vi "EnFlo_Hub.vi"() -> ()   [LabVIEW 2012]
uses:
  Anemometry Sub Vis/Controls/Launch_controls/Open_Calib.ctl
  Anemometry Sub Vis/Controls/Launch_controls/Open_Meas.ctl
  Anemometry Sub Vis/Controls/Launch_controls/Open_Enter_Temp.ctl
  Anemometry Sub Vis/Controls/Launch_controls/Multi_Run_Prog.ctl
  Anemometry Sub Vis/Controls/Launch_controls/EnFlo_arm.ctl
  Anemometry Sub Vis/Controls/Launch_controls/Fast_FID_Valve.ctl
  Anemometry Sub Vis/Controls/Launch_controls/Disp_Setup.ctl
  Anemometry Sub Vis/Controls/Launch_controls/EnFlo_Tun_Setup.ctl
  Anemometry Sub Vis/Controls/Launch_controls/User_Metadata.ctl
  Anemometry Sub Vis/Controls/Launch_controls/Trav_3D_move.ctl
  Anemometry Sub Vis/Controls/Launch_controls/Trav_Space.ctl
  Anemometry Sub Vis/Controls/Launch_controls/Tunnel_speed.ctl
  Anemometry Sub Vis/Controls/Launch_controls/Client_source_control.ctl
  Anemometry Sub Vis/Controls/Launch_controls/Hydrosonic_Manual.ctl
  Anemometry Sub Vis/Controls/Launch_controls/Preference_Panel.ctl
  Anemometry Sub Vis/Controls/Launch_controls/Hot_wire_Calculator.ctl
  Anemometry Sub Vis/Controls/Launch_controls/RW_X_Parker_Config.ctl
  Anemometry Sub Vis/Controls/Launch_controls/LDA_Alignment.ctl
  Anemometry Sub Vis/Controls/Launch_controls/Named_Serial_Comms.ctl
  Anemometry Sub Vis/Controls/Launch_controls/BSA_data_rates.ctl
  Anemometry Sub Vis/Controls/Launch_controls/Serial_Setup.ctl
  Anemometry Sub Vis/Controls/Launch_controls/Post_Process_icon.ctl
  Anemometry Sub Vis/Controls/Launch_controls/Edit_Ascii_file.ctl
  Anemometry Sub Vis/Controls/Launch_controls/Edit_Raw_DF.ctl
  Anemometry Sub Vis/Controls/Launch_controls/Results_file_plotter.ctl
  Anemometry Sub Vis/Controls/Launch_controls/Serial_Port_Names.ctl
  Anemometry Sub Vis/Controls/Launch_controls/Paul.ctl
  Anemometry Sub Vis/Controls/Launch_controls/Tom.ctl
  Anemometry Sub Vis/Controls/Launch_controls/Scani_Valve.ctl
  Anemometry Sub Vis/Controls/Launch_controls/Edit_sever_Channel.ctl
  Anemometry Sub Vis/Controls/Launch_controls/Day_file_plotter.ctl
  Anemometry Sub Vis/Controls/Launch_controls/Plot_Sever_Data.ctl
  Anemometry Sub Vis/Controls/Launch_controls/Adam_Table.ctl
  Anemometry Sub Vis/Controls/Launch_controls/Active_Channel_Control.ctl
  Anemometry Sub Vis/Controls/Setup.ctl
  Anemometry Sub Vis/Controls/Post_Process.ctl
  Anemometry Sub Vis/Controls/Preference_Mode.ctl
  Anemometry Sub Vis/Gen Trav/Trav_mode.ctl
  Anemometry Sub Vis/Controls/User_Specific_mode.ctl
  Anemometry Sub Vis/File/Setup_Filetype.ctl
  Anemometry Sub Vis/Calibration/Calib_mode.ctl
  Anemometry Sub Vis/Controls/Server_Comms.ctl
  Anemometry Sub Vis/Controls/App_Global.ctl
  Anemometry Sub Vis/Globals/Dynamic_call_global.ph.vi
  Anemometry Sub Vis/Globals/Constants_global.vi
  Anemometry Sub Vis/Globals/Preference_global.vi
  Anemometry Sub Vis/Globals/Meas_global.vi
  <vilib>/Platform/browser.llb/Open URL in Default Browser (string).vi
  Anemometry Sub Vis/Globals/Trav_pos_global.vi
  Anemometry Sub Vis/Acquisition/PWA/PWAtasksGLOBAL.vi
  Anemometry Sub Vis/Utilities/Email_transfer_global.vi
panel:
  out "List of ADAM channels to view":string[](array[string])
  out "List of ADAM control channels":string[](array[string])
  out "Analogue Dev Name":string="Dev2"
  out "Numeric":i32
  out "Rig Name":string="EnFlo Tunnel"
  out "All Users":path=path "/System Folder/Preferences/LabVIEW (EnFlo specific)/Meas Setups"
  out "Dummy Measurement":bool
  in  "stop":bool
  in  "Tab Control":T1(tab)
  in  "Tunnel Speed Control":T2
  in  "Traverse Space":T3
  in  "Trav 3D Move":T4 caption="3D Traverse Move"
  in  "User Metadata":T5
  in  "Multi Run Prog":T6
  in  "Enter Temp_Press":T7
  in  "Measurement Prog":T8 caption="Measurement"
  in  "Calibration Prog":T9 caption="Calibration"
  in  "Scani Valve":T10
  in  "LDA Alignment":T11
  in  "Hydrosonic Control":T12
  in  "Fast FID Valve":T13
  in  "Source Control":T14
  in  "Gas Release Setup":T15
  in  "EnFlo Tunnel Setup":T16
  in  "Heater Setup":bool caption="Inlet heater File"
  in  "EnFlo Arm":T17
  in  "EnFlo Tun Display":bool
  in  "Rig_Control":cluster{"Ch Name":string, "Boolean":bool}[](array[cluster])
  in  "ADAM Channels Control":T18 caption="Change Active Channels"
  in  "ADAM Scan Table":T19 caption="Run ADAM Scan Table"
  in  "Edit Server Channel":T20
  in  "Plot Server Channels":T21 caption="Plot Server Data"
  in  "Day Files Plotter":T22 caption="Plot Data From File"
  out "Current Values":cluster{"Ch Name":string, "Numeric":dbl}[](array[cluster])
  in  "Results File Plotter":T23
  in  "Edit Raw Data Files":T24
  in  "Edit ASCII File":T25
  in  "Post Process Raw Data":T26
  in  "Port Names":T27
  in  "Serial Setup":T28
  in  "LDA Data Rate":T29
  in  "Named Serial Comms":T30
  in  "RW Trav Setup":T31
  in  "Hot Wire Calc":T32
  in  "Preference Panel":T33
  in  "Tom Lawton t.lawton@surrey.ac.uk":T34 caption="For hardware support"
  in  "Paul Hayden p.hayden@surrey.ac.uk":T35 caption="For software support"
  in  "Online Manual":bool
  out "VI Name":string
  out "Iterations":i32
  # "Or give us a call on Tel: 01483 689545"
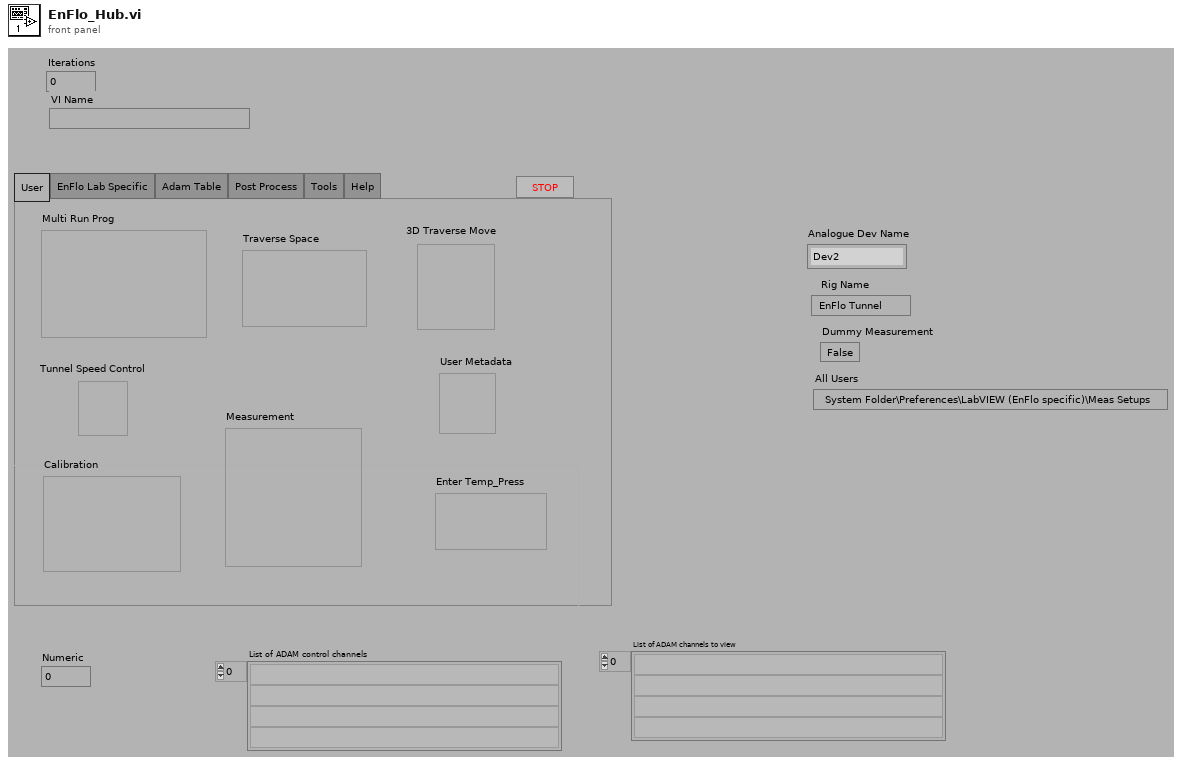
[diagram p1: front panel]
types:
  T1 = enum32{"User", "EnFlo Lab Specific", "Adam Table", "Post Process", "Tools", "Help"}
  T2 = typedef "Tunnel_speed.ctl" = bool
  T3 = typedef "Trav_Space.ctl" = bool
  T4 = typedef "Trav_3D_move.ctl" = bool
  T5 = typedef "User_Metadata.ctl" = bool
  T6 = typedef "Multi_Run_Prog.ctl" = bool
  T7 = typedef "Open_Enter_Temp.ctl" = bool
  T8 = typedef "Open_Meas.ctl" = bool
  T9 = typedef "Open_Calib.ctl" = bool
  T10 = typedef "Scani_Valve.ctl" = bool
  T11 = typedef "LDA_Alignment.ctl" = bool
  T12 = typedef "Hydrosonic_Manual.ctl" = bool
  T13 = typedef "Fast_FID_Valve.ctl" = bool
  T14 = typedef "Client_source_control.ctl" = bool
  T15 = typedef "Disp_Setup.ctl" = bool
  T16 = typedef "EnFlo_Tun_Setup.ctl" = bool
  T17 = typedef "EnFlo_arm.ctl" = bool
  T18 = typedef "Active_Channel_Control.ctl" = bool
  T19 = typedef "Adam_Table.ctl" = bool
  T20 = typedef "Edit_sever_Channel.ctl" = bool
  T21 = typedef "Plot_Sever_Data.ctl" = bool
  T22 = typedef "Day_file_plotter.ctl" = bool
  T23 = typedef "Results_file_plotter.ctl" = bool
  T24 = typedef "Edit_Raw_DF.ctl" = bool
  T25 = typedef "Edit_Ascii_file.ctl" = bool
  T26 = typedef "Post_Process_icon.ctl" = bool
  T27 = typedef "Serial_Port_Names.ctl" = bool
  T28 = typedef "Serial_Setup.ctl" = bool
  T29 = typedef "BSA_data_rates.ctl" = bool
  T30 = typedef "Named_Serial_Comms.ctl" = bool
  T31 = typedef "RW_X_Parker_Config.ctl" = bool
  T32 = typedef "Hot_wire_Calculator.ctl" = bool
  T33 = typedef "Preference_Panel.ctl" = bool
  T34 = typedef "Tom.ctl" = bool
  T35 = typedef "Paul.ctl" = bool
  T36 = typedef "Post_Process.ctl" = enum16{"Take New Data", "Post Process Raw Data File"}
  T37 = typedef "Setup.ctl" = enum16{"Run Program", "Show Setup", "Save Current Setup", "Setup Front Panel"}
  T38 = enum16{"Get Channel Names", "Get Current Value", "Update Channel Value", "Update Channel Description"}
  T39 = enum32{"Invalid", "Standard", "Closed", "Hidden", "Minimized", "Maximized"}
  T40 = typedef "Preference_Mode.ctl" = enum16{"Load Preferences from file", "Save Preferences to file", "Load, Edit then Save"}
  T41 = typedef "User_Specific_mode.ctl" = enum16{"Check VI only", "Run VI"}
  T42 = typedef "Trav_mode.ctl" = enum16{"Move traverse", "Read traverse position", "Teach Position"}
  T43 = typedef "Setup_Filetype.ctl" = enum16{"Measurement Setups", "Calibration Setups", "General", "Results File Plotter Setups", "Speed Calib Tweaks"}
  T44 = enum16{"Load Command File", "Save Command File", "Check Multi Run Prog", "Check Multi Run Prog With Live Moves", "Run Multi Run Prog"}
  T45 = typedef "Calib_mode.ctl" = enum16{"Show Setup", "Take a New Calibration Point", "Refit Curve", "Setup Front Panel"}
  T46 = typedef "Tunnel_Coordinates.ctl" = enum16{"Work in Tunnel Coordinates", "Work in Model Coordinates"}
  T47 = typedef "App_Global.ctl" = enum16{"Read Global", "Write to Global", "Initialise Array"}
  T48 = typedef "App_Ref_Cluster.ctl" = cluster{"Server IP & Port No":string, "Application reference":refnum<vi>}
  T49 = typedef "Server_Comms.ctl" = enum16{"Server Link Healthy", "Do Not Link To Server"}
  T50 = typedef "Ch_description_ADAM.ctl" = cluster{"Ch Name":string, "Type":T51, "Function":T52, "Ch State":T53, "Calibration type":T54, "A":dbl, "B":dbl, "C":dbl, "D":dbl, "Comments":string, "Address":T55, "String":string, "Duty":u16}
  T51 = typedef "Module_type_ADAM.ctl" = string
  T52 = typedef "Function_ADAM.ctl" = enum16{"Analogue Input", "Digital Input", "Event counter", "Event rate", "Analogue Output", "Digital Output", "Relay Output"}
  T53 = typedef "Channel_State.ctl" = enum16{"On", "Off", "Always On", "Always Off"}
  T54 = typedef "Calib_type_ADAM.ctl" = enum16{"Raw", "Bx + A", "Cx^2 + Bx + A", "Dx^3 + Cx^2 + Bx + A", "In Band", "Hi-Tec Q", "Hi-Tec M_dot", "Text"}
  T55 = typedef "Address.ctl" = cluster{"Main":i32, "Ch.":i32, "Sub":i32, "Port Name":string}
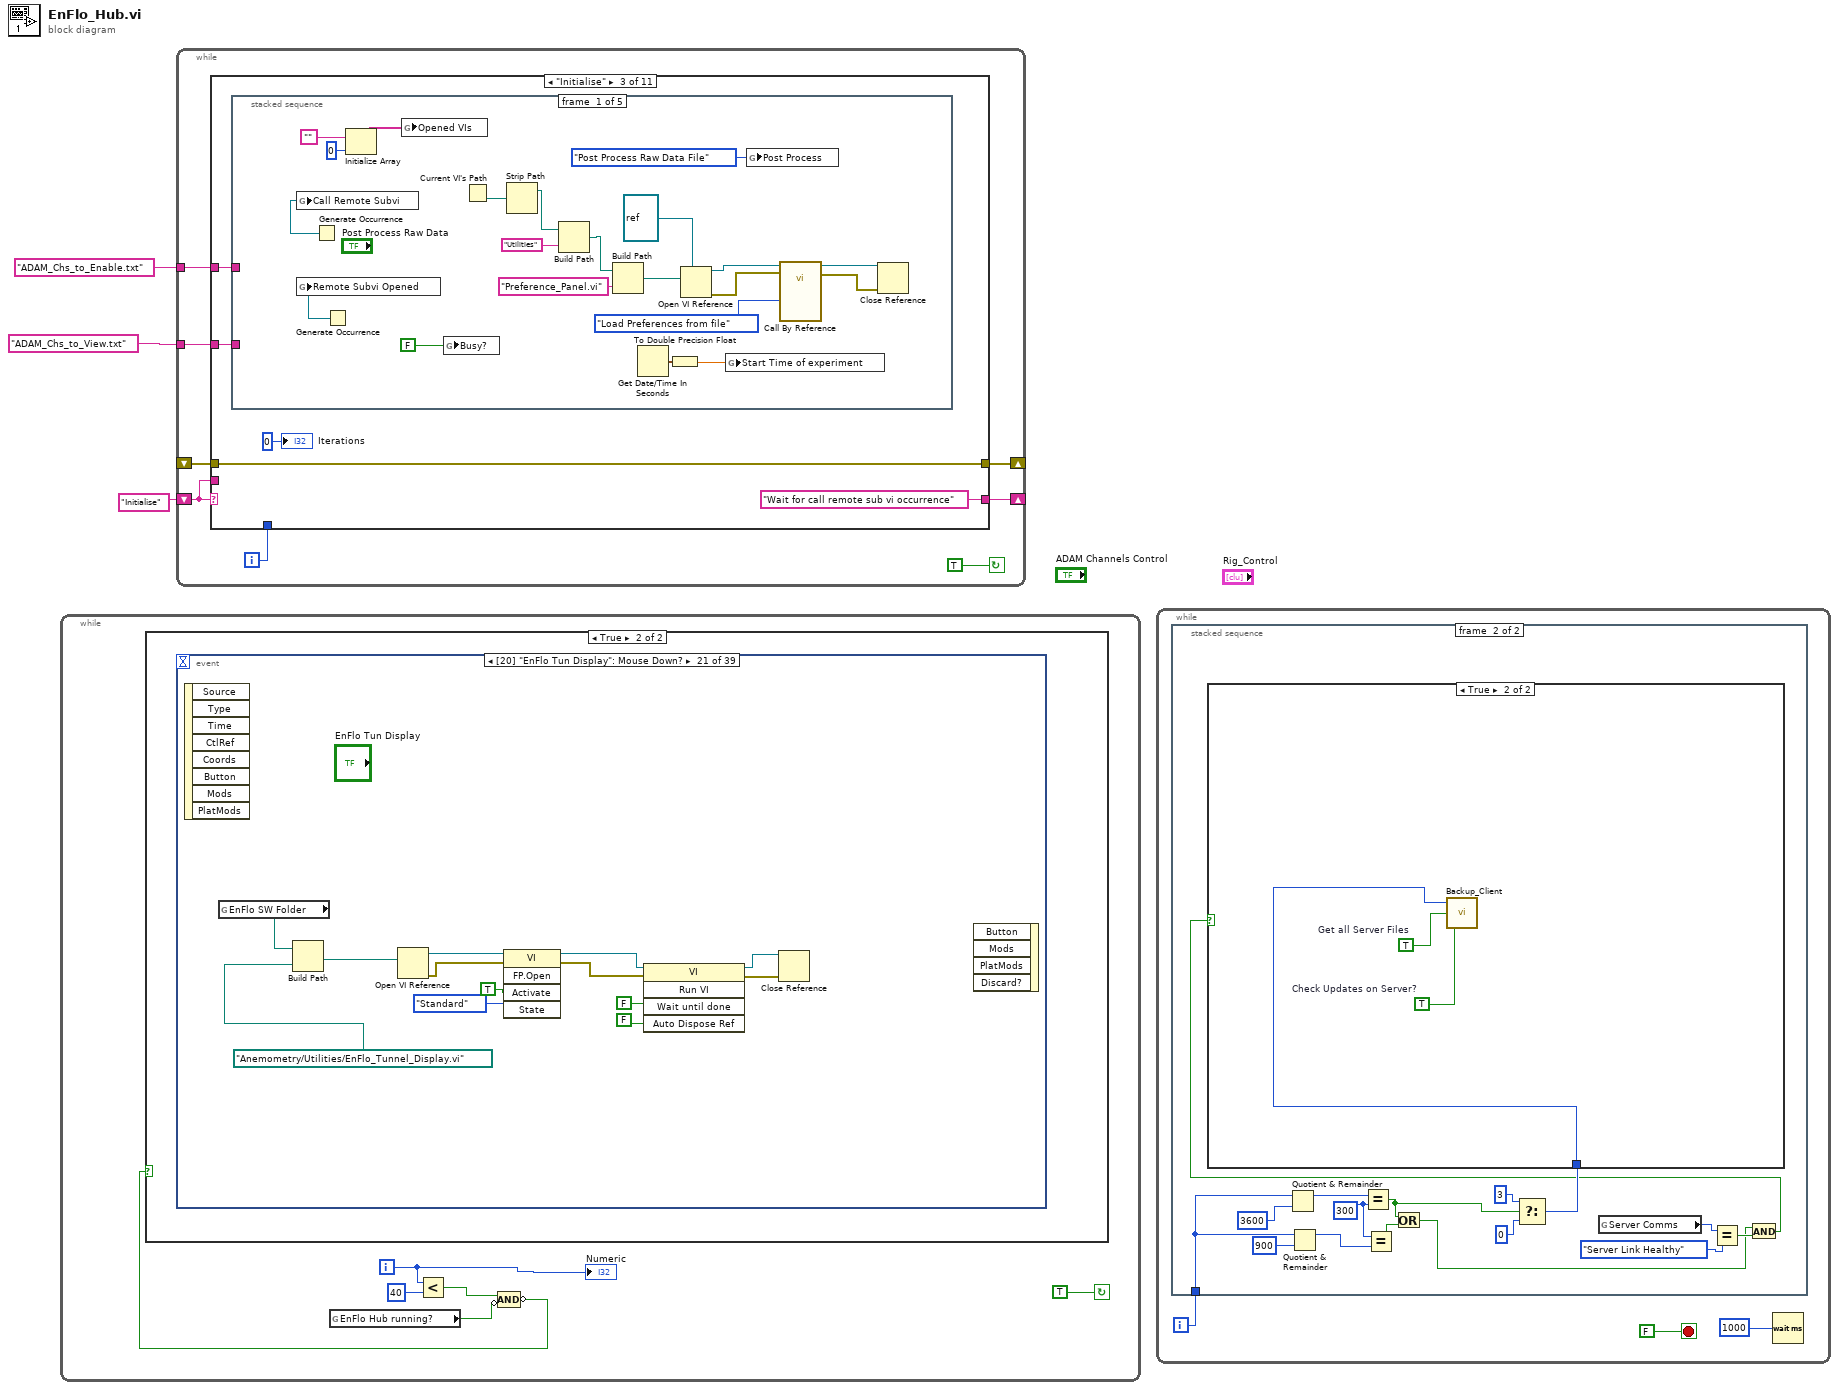
[diagram p0: block diagram]
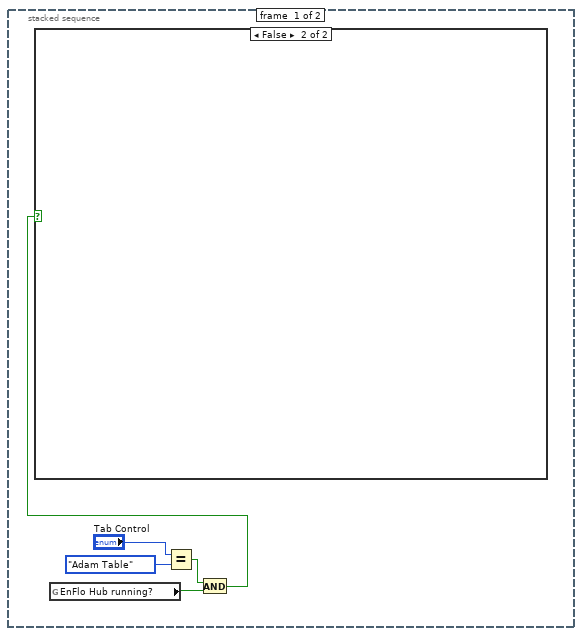
[diagram p2: hidden frame]
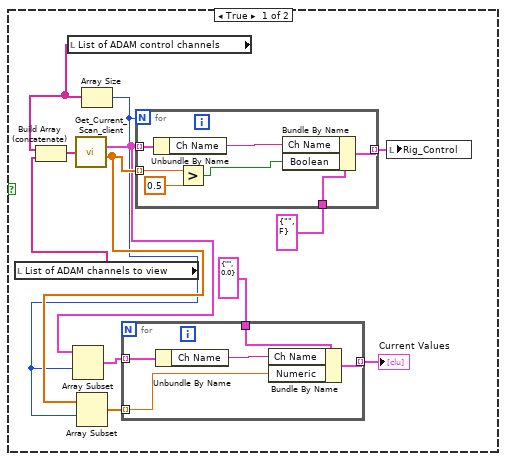
[diagram p3: hidden frame]
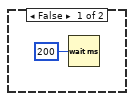
[diagram p5: hidden frame]
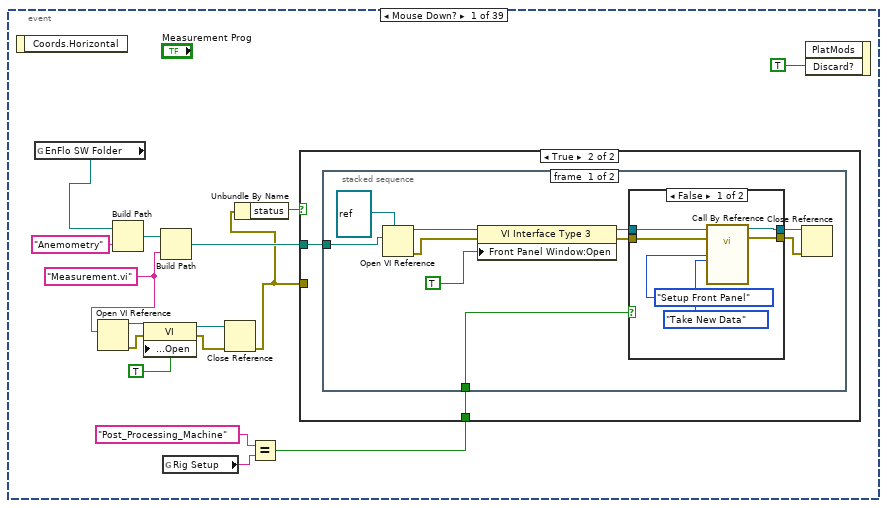
[diagram p6: hidden frame]
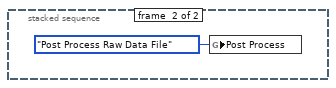
[diagram p9: hidden frame]
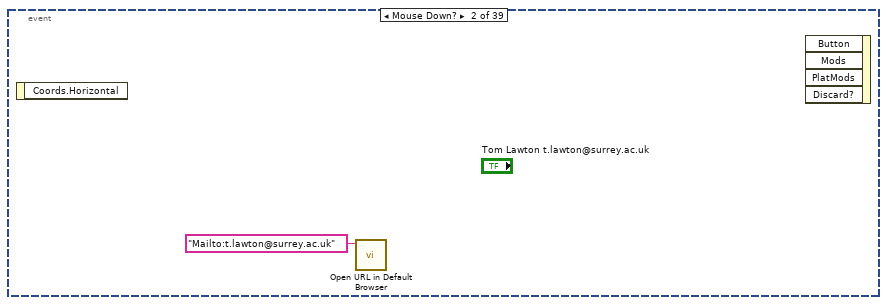
[diagram p10: hidden frame]
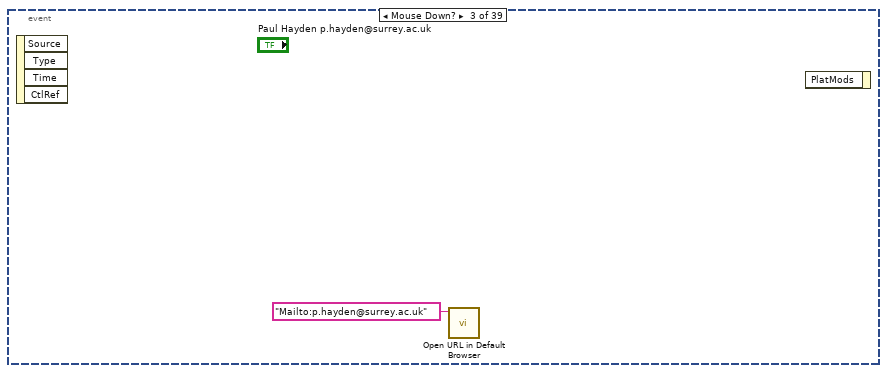
[diagram p11: hidden frame]
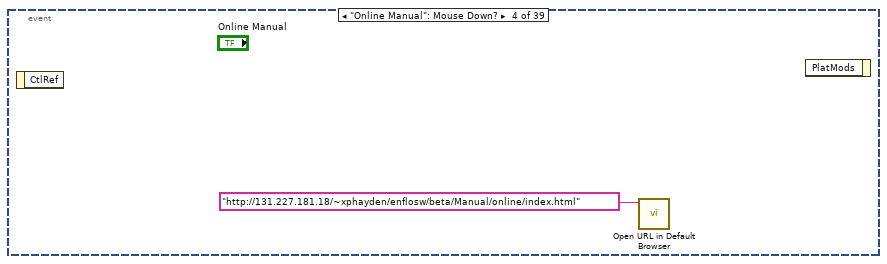
[diagram p12: hidden frame]
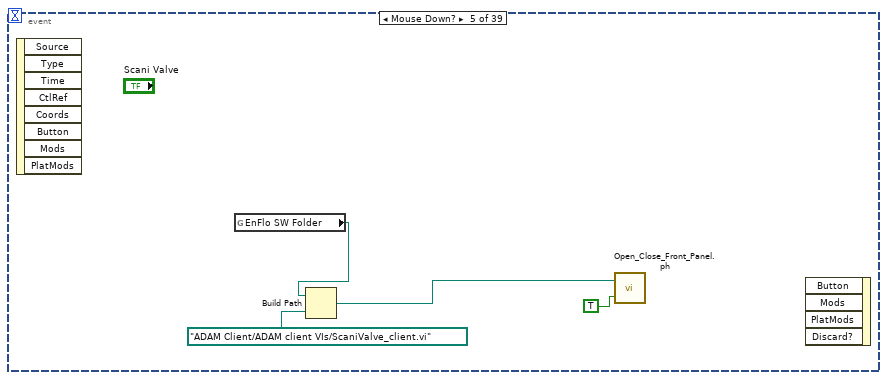
[diagram p13: hidden frame]
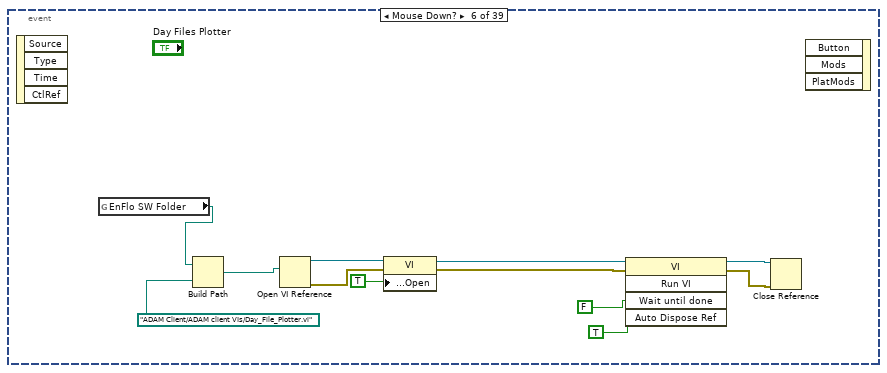
[diagram p14: hidden frame]
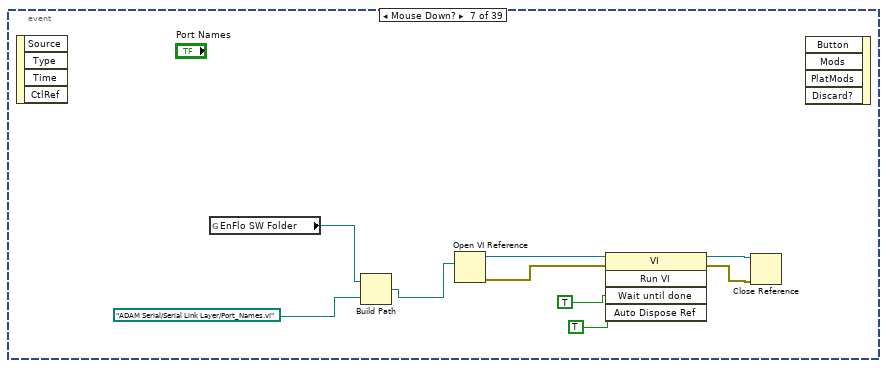
[diagram p15: hidden frame]
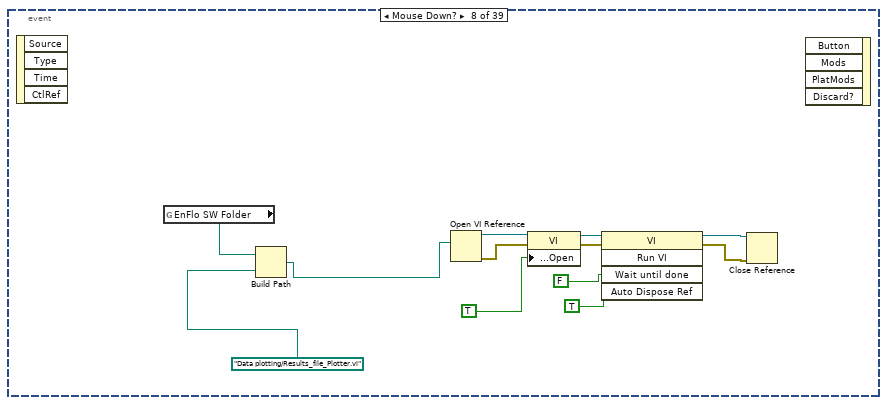
[diagram p16: hidden frame]
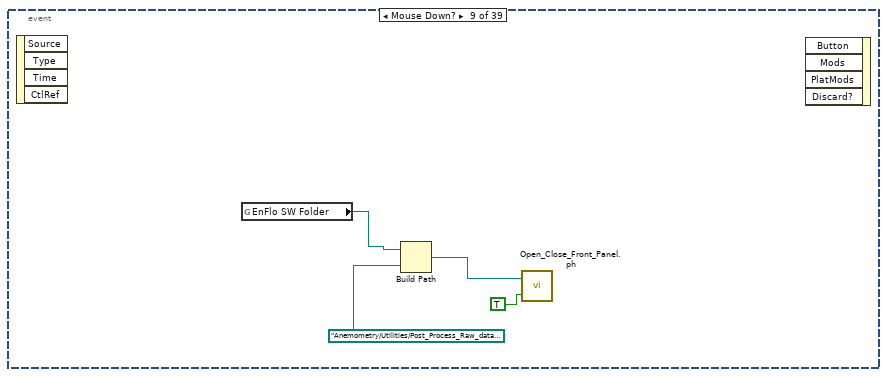
[diagram p17: hidden frame]
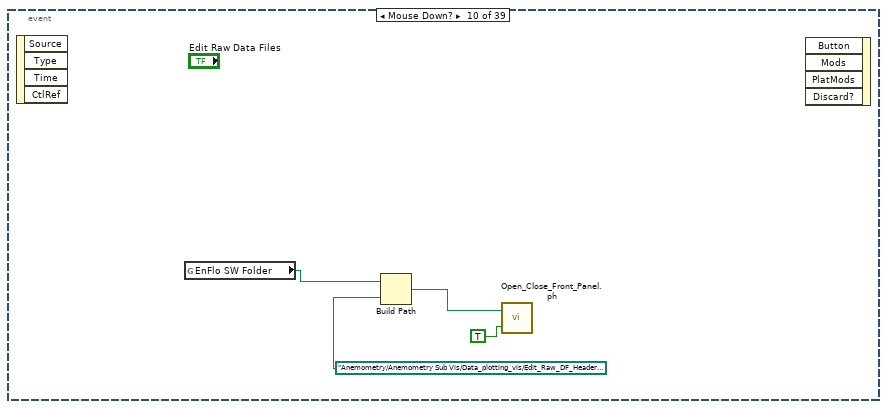
[diagram p18: hidden frame]
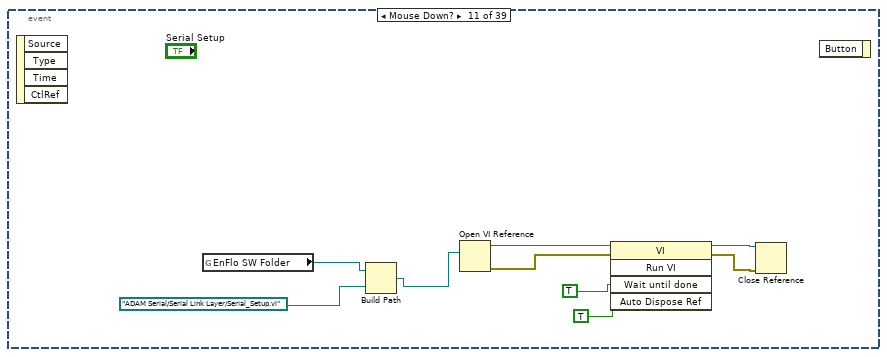
[diagram p19: hidden frame]
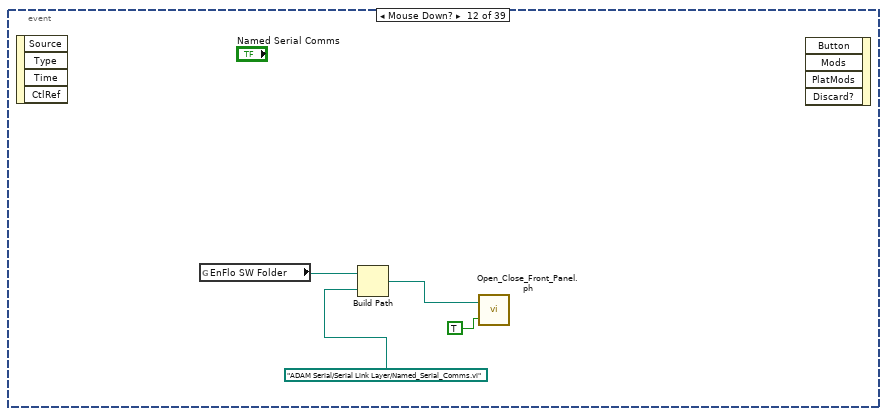
[diagram p20: hidden frame]
diagram:
  n1 = while {
    i -> [w8]
    stop <- TRUE continue-if-true
    n2 = global read "Dynamic_call_global.ph.vi" "EnFlo Hub running?"() -> (w6:bool)
    n3 = Less?(x=w8, y=40) -> (x < y?=w5:bool)
    n4 = Compound Arithmetic op=AND(w5, invert w6) -> (invert w4:bool)
    n5 = case shown="True" w4 {
      frame False {
        n6 = Wait (ms)(milliseconds to wait=u32 200) -> ()  [unwired: 1 out]
      }
      frame True {
        n7 = event shown="[20] \"EnFlo Tun Display\": Mouse Down?" {
          selector: _ -> [_ _ _ _ _ _ _ _ _ _ _ _ _ _ _ _ _ _ _ _ _ _ _ _ _ _ _ _ _ _ _ _ _ _ _ _ _ _ _]
          dyn-events: _ -> [_ _ _ _ _ _ _ _ _ _ _ _ _ _ _ _ _ _ _ _ _ _ _ _ _ _ _ _ _ _ _ _ _ _ _ _ _ _ _]
          timeout: _ -> [_ _ _ _ _ _ _ _ _ _ _ _ _ _ _ _ _ _ _ _ _ _ _ _ _ _ _ _ _ _ _ _ _ _ _ _ _ _ _]
          event Mouse Down? {
            w19 = "Measurement.vi" ("name or relative path")
            n8 = event-data() -> ()  [unwired: 2 out]
            n9 = global read "Constants_global.vi" "EnFlo SW Folder"() -> (w22:path)
            n10 = Open VI Reference(vi path=w19) -> (vi reference=w18:refnum<vi>, error out=w17:errorcluster)  [unwired: 1 in, 4 out]
            n11 = Build Path(base path=w22, name or relative path="Anemometry") -> (appended path=w25:path)
            n12 = property class="VI"(reference=w18, error in=w17, "Front Panel Window:Open"=TRUE) -> (reference out=w15:refnum<vi>, error out=w16:errorcluster)
            n13 = Build Path(base path=w25, name or relative path=w19) -> (appended path=w23:path)
            n14 = global read "Preference_global.vi" "Rig Setup"() -> (w13:string)
            n15 = Close Reference(reference=w15, error in (no error)=w16) -> (error out=w14:errorcluster)
            n16 = Unbundle By Name(w14) -> ("status"=w24:bool)
            n17 = Equal?(x="Post_Processing_Machine" ("Rig Setup"), y=w13) -> (x = y?=w11:bool)
            n18 = case shown="True" w24 {
              tunnel: w23 -> [_ w28]
              tunnel: w14 -> [_ _]
              tunnel: w11 -> [_ w27]
              frame False {
              }
              frame True {
                n19 = stacked-sequence {
                  tunnel: w28 -> [w38 _]
                  tunnel: w27 -> [w29 _]
                  frame #0 {
                    n20 = Open VI Reference(type specifier VI Refnum (for type only)=refnum<vi> refnum, vi path=w38) -> (vi reference=w36:refnum<vi>, error out=w35:errorcluster)  [unwired: 1 in, 3 out]
                    n21 = property class="VI Interface Type 3"(reference=w36, error in=w35, "Front Panel Window:Open"=TRUE) -> (reference out=w31:refnum<vi>, error out=w30:errorcluster)
                    n22 = case shown="False" w29 {
                      tunnel: [w44 w46] -> w34
                      tunnel: [w43 w45] -> w33
                      tunnel: w31 -> [w42 w46]
                      tunnel: w30 -> [w41 w45]
                      frame False {
                        n23 = call-by-ref "?"(reference=w42, error in=w41, "setup"=Setup."Setup Front Panel", "Post Process"=Post_Process."Take New Data") -> (reference out=w44:refnum<vi>, error out=w43:errorcluster)  [unwired: 16 in, 2 out]
                      }
                      frame True {
                      }
                    }
                    n24 = Close Reference(reference=w34, error in (no error)=w33) -> ()  [unwired: 1 out]
                  }
                  frame #1 {
                    n25 = global write "Meas_global.vi" "Post Process"(Post_Process."Post Process Raw Data File" ("Post Process")) -> ()
                  }
                }
              }
            }
            n26 = event-data("Discard?"=TRUE) -> ()  [unwired: 1 in, 2 out]
          }
          event Mouse Down? {
            n27 = event-data() -> ()  [unwired: 2 out]
            n28 = call-poly <vilib>:"Open URL in Default Browser.vi"("URL"="Mailto:t.lawton@surrey.ac.uk") -> ()  [unwired: 1 in, 6 out]
            n29 = event-data() -> ()  [unwired: 1 in, 5 out]
          }
          event Mouse Down? {
            n30 = event-data() -> ()  [unwired: 5 out]
            n31 = call-poly <vilib>:"Open URL in Default Browser.vi"("URL"="Mailto:p.hayden@surrey.ac.uk") -> ()  [unwired: 1 in, 6 out]
            n32 = event-data() -> ()  [unwired: 1 in, 2 out]
          }
          event "Online Manual": Mouse Down? {
            n33 = event-data() -> ()  [unwired: 2 out]
            n34 = call-poly <vilib>:"Open URL in Default Browser.vi"("URL"="http://131.227.181.18/~xphayden/enflosw/beta/Manual/online/index.html") -> ()  [unwired: 1 in, 6 out]
            n35 = event-data() -> ()  [unwired: 1 in, 2 out]
          }
          event Mouse Down? {
            n36 = event-data() -> ()  [unwired: 9 out]
            n37 = global read "Constants_global.vi" "EnFlo SW Folder"() -> (w51:path)
            n38 = Build Path(base path=w51, name or relative path=path "ADAM Client/ADAM client VIs/ScaniValve_client.vi") -> (appended path=w54:path)
            n39 = call "Open_Close_Front_Panel.ph.vi"("Front Panel Window:Open"=TRUE, "VI path"=w54) -> ()  [unwired: 2 out]
            n40 = event-data() -> ()  [unwired: 1 in, 5 out]
          }
          event Mouse Down? {
            n41 = event-data() -> ()  [unwired: 5 out]
            n42 = global read "Constants_global.vi" "EnFlo SW Folder"() -> (w55:path)
            n43 = Build Path(base path=w55, name or relative path=path "ADAM Client/ADAM client VIs/Day_File_Plotter.vi") -> (appended path=w61:path)
            n44 = Open VI Reference(vi path=w61) -> (vi reference=w62:refnum<vi>, error out=w64:errorcluster)  [unwired: 2 in, 3 out]
            n45 = property class="VI"(reference=w62, error in=w64, "Front Panel Window:Open"=TRUE) -> (reference out=w66:refnum<vi>, error out=w65:errorcluster)
            n46 = invoke class="VI" method="Run VI"(reference=w66, error in=w65, "Wait until done"=FALSE, "Auto Dispose Ref"=TRUE) -> (reference out=w57:refnum<vi>, error out=w58:errorcluster)  [unwired: 1 in, 3 out]
            n47 = Close Reference(reference=w57, error in (no error)=w58) -> ()  [unwired: 1 out]
            n48 = event-data() -> ()  [unwired: 1 in, 4 out]
          }
          event Mouse Down? {
            n49 = event-data() -> ()  [unwired: 5 out]
            n50 = global read "Constants_global.vi" "EnFlo SW Folder"() -> (w67:path)
            n51 = Build Path(base path=w67, name or relative path=path "ADAM Serial/Serial Link Layer/Port_Names.vi") -> (appended path=w69:path)
            n52 = Open VI Reference(vi path=w69) -> (vi reference=w74:refnum<vi>, error out=w75:errorcluster)  [unwired: 1 in, 4 out]
            n53 = invoke class="VI" method="Run VI"(reference=w74, error in=w75, "Wait until done"=TRUE, "Auto Dispose Ref"=TRUE) -> (reference out=w70:refnum<vi>, error out=w71:errorcluster)  [unwired: 1 in, 3 out]
            n54 = Close Reference(reference=w70, error in (no error)=w71) -> ()  [unwired: 1 out]
            n55 = event-data() -> ()  [unwired: 1 in, 5 out]
          }
          event Mouse Down? {
            n56 = event-data() -> ()  [unwired: 5 out]
            n57 = global read "Constants_global.vi" "EnFlo SW Folder"() -> (w76:path)
            n58 = Build Path(base path=w76, name or relative path=path "Data plotting/Results_file_Plotter.vi") -> (appended path=w79:path)
            n59 = Open VI Reference(vi path=w79) -> (vi reference=w81:refnum<vi>, error out=w78:errorcluster)  [unwired: 1 in, 4 out]
            n60 = property class="VI"(reference=w81, error in=w78, "Front Panel Window:Open"=TRUE) -> (reference out=w82:refnum<vi>, error out=w83:errorcluster)
            n61 = invoke class="VI" method="Run VI"(reference=w82, error in=w83, "Wait until done"=FALSE, "Auto Dispose Ref"=TRUE) -> (reference out=w84:refnum<vi>, error out=w85:errorcluster)  [unwired: 1 in, 3 out]
            n62 = Close Reference(reference=w84, error in (no error)=w85) -> ()  [unwired: 1 out]
            n63 = event-data() -> ()  [unwired: 1 in, 5 out]
          }
          event Mouse Down? {
            n64 = event-data() -> ()  [unwired: 5 out]
            n65 = global read "Constants_global.vi" "EnFlo SW Folder"() -> (w88:path)
            n66 = Build Path(base path=w88, name or relative path=path "Anemometry/Utilities/Post_Process_Raw_data.vi") -> (appended path=w90:path)
            n67 = call "Open_Close_Front_Panel.ph.vi"("Front Panel Window:Open"=TRUE, "VI path"=w90) -> ()  [unwired: 2 out]
            n68 = event-data() -> ()  [unwired: 1 in, 5 out]
          }
          event Mouse Down? {
            n69 = event-data() -> ()  [unwired: 5 out]
            n70 = global read "Constants_global.vi" "EnFlo SW Folder"() -> (w92:path)
            n71 = Build Path(base path=w92, name or relative path=path "Anemometry/Anemometry Sub Vis/Data_plotting_vis/Edit_Raw_DF_Header.vi") -> (appended path=w94:path)
            n72 = call "Open_Close_Front_Panel.ph.vi"("Front Panel Window:Open"=TRUE, "VI path"=w94) -> ()  [unwired: 2 out]
            n73 = event-data() -> ()  [unwired: 1 in, 5 out]
          }
          event Mouse Down? {
            n74 = event-data() -> ()  [unwired: 5 out]
            n75 = global read "Constants_global.vi" "EnFlo SW Folder"() -> (w96:path)
            n76 = Build Path(base path=w96, name or relative path=path "ADAM Serial/Serial Link Layer/Serial_Setup.vi") -> (appended path=w98:path)
            n77 = Open VI Reference(vi path=w98) -> (vi reference=w103:refnum<vi>, error out=w104:errorcluster)  [unwired: 1 in, 4 out]
            n78 = invoke class="VI" method="Run VI"(reference=w103, error in=w104, "Wait until done"=TRUE, "Auto Dispose Ref"=TRUE) -> (reference out=w99:refnum<vi>, error out=w100:errorcluster)  [unwired: 1 in, 3 out]
            n79 = Close Reference(reference=w99, error in (no error)=w100) -> ()  [unwired: 1 out]
            n80 = event-data() -> ()  [unwired: 1 in, 2 out]
          }
          event Mouse Down? {
            n81 = event-data() -> ()  [unwired: 5 out]
            n82 = global read "Constants_global.vi" "EnFlo SW Folder"() -> (w106:path)
            n83 = Build Path(base path=w106, name or relative path=path "ADAM Serial/Serial Link Layer/Named_Serial_Comms.vi") -> (appended path=w108:path)
            n84 = call "Open_Close_Front_Panel.ph.vi"("Front Panel Window:Open"=TRUE, "VI path"=w108) -> ()  [unwired: 2 out]
            n85 = event-data() -> ()  [unwired: 1 in, 5 out]
          }
          event Mouse Down? {
            n86 = event-data() -> ()  [unwired: 5 out]
            n87 = global read "Constants_global.vi" "EnFlo SW Folder"() -> (w109:path)
            n88 = Build Path(base path=w109, name or relative path=path "Anemometry/Anemometry Sub Vis/LDA/LDA_data_rate.vi") -> (appended path=w111:path)
            n89 = call "Open_Close_Front_Panel.ph.vi"("Front Panel Window:Open"=TRUE, "VI path"=w111) -> ()  [unwired: 2 out]
            n90 = event-data() -> ()  [unwired: 1 in, 2 out]
          }
          event Mouse Down? {
            n91 = event-data() -> ()  [unwired: 5 out]
            n92 = global read "Constants_global.vi" "EnFlo SW Folder"() -> (w123:path)
            n93 = Build Path(base path=w123, name or relative path=path "ADAM Client/ADAM client VIs/Control_Channel_Status.vi") -> (appended path=w113:path)
            n94 = Open VI Reference(vi path=w113) -> (vi reference=w116:refnum<vi>, error out=w114:errorcluster)  [unwired: 1 in, 4 out]
            n95 = property class="VI"(reference=w116, error in=w114, "Front Panel Window:Open"=TRUE) -> (reference out=w117:refnum<vi>, error out=w118:errorcluster)
            n96 = invoke class="VI" method="Run VI"(reference=w117, error in=w118, "Wait until done"=FALSE, "Auto Dispose Ref"=TRUE) -> (reference out=w119:refnum<vi>, error out=w120:errorcluster)  [unwired: 1 in, 3 out]
            n97 = Close Reference(reference=w119, error in (no error)=w120) -> ()  [unwired: 1 out]
            n98 = event-data() -> ()  [unwired: 1 in, 2 out]
          }
          event Mouse Down? {
            n99 = event-data() -> ()  [unwired: 5 out]
            n100 = global read "Constants_global.vi" "EnFlo SW Folder"() -> (w125:path)
            n101 = Build Path(base path=w125, name or relative path=path "Anemometry/Utilities/LDA_Beam_Alignment.vi") -> (appended path=w127:path)
            n102 = call "Open_Close_Front_Panel.ph.vi"("Front Panel Window:Open"=TRUE, "VI path"=w127) -> ()  [unwired: 2 out]
            n103 = event-data() -> ()  [unwired: 1 in, 5 out]
          }
          event Mouse Down? {
            w130 = FALSE  # Wait until done
            n104 = event-data() -> ()  [unwired: 5 out]
            n105 = call "Run_Enter_Temp.vi"("Wait until done"=w130) -> ()  [unwired: 1 out]
            n106 = event-data("Discard?"=TRUE) -> ()  [unwired: 1 in, 4 out]
          }
          event Mouse Down? {
            n107 = event-data() -> ()  [unwired: 5 out]
            n108 = global read "Constants_global.vi" "EnFlo SW Folder"() -> (w131:path)
            n109 = Build Path(base path=w131, name or relative path=path "Anemometry/Utilities/Edit_ASCI_file.vi") -> (appended path=w134:path)
            n110 = call "Open_Close_Front_Panel.ph.vi"("Front Panel Window:Open"=TRUE, "VI path"=w134) -> ()  [unwired: 2 out]
            n111 = event-data() -> ()  [unwired: 1 in, 5 out]
          }
          event "Heater Setup": Mouse Down? {
            n112 = event-data() -> ()  [unwired: 5 out]
            n113 = global read "Constants_global.vi" "EnFlo SW Folder"() -> (w135:path)
            n114 = Build Path(base path=w135, name or relative path=path "Anemometry/Utilities/Create_Heater_Setpoints_File.vi") -> (appended path=w138:path)
            n115 = call "Open_Close_Front_Panel.ph.vi"("Front Panel Window:Open"=TRUE, "VI path"=w138) -> ()  [unwired: 2 out]
            n116 = event-data() -> ()  [unwired: 1 in, 5 out]
          }
          event Mouse Down? {
            n117 = event-data() -> ()  [unwired: 5 out]
            n118 = global read "Constants_global.vi" "EnFlo SW Folder"() -> (w139:path)
            n119 = Build Path(base path=w139, name or relative path=path "ADAM Client/Sub VIs/Gas_Release_Control.vi") -> (appended path=w142:path)
            n120 = call "Open_Close_Front_Panel.ph.vi"("Front Panel Window:Open"=TRUE, "VI path"=w142) -> ()  [unwired: 2 out]
            n121 = event-data() -> ()  [unwired: 1 in, 5 out]
          }
          event Mouse Down? {
            n122 = event-data() -> ()  [unwired: 5 out]
            n123 = global read "Constants_global.vi" "EnFlo SW Folder"() -> (w143:path)
            n124 = Build Path(base path=w143, name or relative path=path "ADAM Client/ADAM client VIs/Edit_Server_Channel.vi") -> (appended path=w153:path)
            n125 = Open VI Reference(type specifier VI Refnum (for type only)=refnum<vi> refnum, vi path=w153) -> (vi reference=w146:refnum<vi>, error out=w147:errorcluster)  [unwired: 1 in, 3 out]
            n126 = property class="VI Interface Type 4"(reference=w146, error in=w147, "Front Panel Window:Open"=TRUE) -> (reference out=w149:refnum<vi>, error out=w150:errorcluster)
            n127 = call-by-ref "?"(reference=w149, error in=w150, "Mode"=T38."Get Channel Names") -> (reference out=w151:refnum<vi>, error out=w152:errorcluster)  [unwired: 5 in]
            n128 = Close Reference(reference=w151, error in (no error)=w152) -> ()  [unwired: 1 out]
            n129 = event-data() -> ()  [unwired: 1 in, 5 out]
          }
          event "EnFlo Tun Display": Mouse Down? {
            n130 = event-data() -> ()  [unwired: 9 out]
            n131 = global read "Constants_global.vi" "EnFlo SW Folder"() -> (w166:path)
            n132 = Build Path(base path=w166, name or relative path=path "Anemometry/Utilities/EnFlo_Tunnel_Display.vi") -> (appended path=w161:path)
            n133 = Open VI Reference(vi path=w161) -> (vi reference=w160:refnum<vi>, error out=w159:errorcluster)  [unwired: 5 in]
            n134 = invoke class="VI" method="FP.Open"(reference=w160, error in=w159, "Activate"=TRUE ("Activate?"), "State"=T39."Standard") -> (reference out=w158:refnum<vi>, error out=w157:errorcluster)  [unwired: 1 in, 3 out]
            n135 = invoke class="VI" method="Run VI"(reference=w158, error in=w157, "Wait until done"=FALSE ("Wait Until Done"), "Auto Dispose Ref"=FALSE ("Wait until done")) -> (reference out=w162:refnum<vi>, error out=w163:errorcluster)  [unwired: 1 in, 3 out]
            n136 = Close Reference(reference=w162, error in (no error)=w163) -> ()  [unwired: 1 out]
            n137 = event-data() -> ()  [unwired: 5 in, 1 out]
          }
          event Mouse Down? {
            n138 = event-data() -> ()  [unwired: 5 out]
            n139 = global read "Constants_global.vi" "EnFlo SW Folder"() -> (w168:path)
            n140 = Build Path(base path=w168, name or relative path=path "ADAM Client/ADAM client VIs/Set_Tunnel_Speed.vi") -> (appended path=w171:path)
            n141 = call "Open_Close_Front_Panel.ph.vi"("Front Panel Window:Open"=TRUE, "VI path"=w171) -> ()  [unwired: 2 out]
            n142 = event-data() -> ()  [unwired: 1 in, 5 out]
          }
          event Mouse Down? {
            n143 = event-data() -> ()  [unwired: 5 out]
            n144 = global read "Constants_global.vi" "EnFlo SW Folder"() -> (w172:path)
            n145 = Build Path(base path=w172, name or relative path=path "ADAM Client/ADAM client VIs/Plot_Server_Data.vi") -> (appended path=w175:path)
            n146 = Open VI Reference(vi path=w175) -> (vi reference=w177:refnum<vi>, error out=w174:errorcluster)  [unwired: 1 in, 4 out]
            n147 = property class="VI"(reference=w177, error in=w174, "Front Panel Window:Open"=TRUE) -> (reference out=w178:refnum<vi>, error out=w179:errorcluster)
            n148 = invoke class="VI" method="Run VI"(reference=w178, error in=w179, "Wait until done"=FALSE, "Auto Dispose Ref"=TRUE) -> (reference out=w180:refnum<vi>, error out=w181:errorcluster)  [unwired: 1 in, 3 out]
            n149 = Close Reference(reference=w180, error in (no error)=w181) -> ()  [unwired: 1 out]
            n150 = event-data() -> ()  [unwired: 1 in, 5 out]
          }
          event Mouse Down? {
            n151 = event-data() -> ()  [unwired: 5 out]
            n152 = Two Button Dialog(message="Are you sure that you want to Run the ADAM Scan table on this machine?", 1:"Run" ("F button name (\"Cancel\")"), 2:"Cancel" ("T button name (\"OK\")")) -> (T button?=w185:bool)
            n153 = case shown="False" w185 {
              frame False {
                n154 = global read "Constants_global.vi" "EnFlo SW Folder"() -> (w188:path)
                n155 = Build Path(base path=w188, name or relative path=path "ADAM Server/ADAM_scan_table.vi") -> (appended path=w191:path)
                n156 = Open VI Reference(vi path=w191) -> (vi reference=w193:refnum<vi>, error out=w190:errorcluster)  [unwired: 1 in, 4 out]
                n157 = property class="VI"(reference=w193, error in=w190, "Front Panel Window:Open"=TRUE) -> (reference out=w194:refnum<vi>, error out=w195:errorcluster)
                n158 = invoke class="VI" method="Run VI"(reference=w194, error in=w195, "Wait until done"=FALSE, "Auto Dispose Ref"=TRUE) -> (reference out=w196:refnum<vi>, error out=w197:errorcluster)  [unwired: 1 in, 3 out]
                n159 = Close Reference(reference=w196, error in (no error)=w197) -> ()  [unwired: 1 out]
              }
              frame True {
              }
            }
            n160 = event-data() -> ()  [unwired: 1 in, 2 out]
          }
          event Mouse Down? {
            n161 = event-data() -> ()  [unwired: 5 out]
            n162 = global read "Constants_global.vi" "EnFlo SW Folder"() -> (w202:path)
            n163 = Build Path(base path=w202, name or relative path=path "ADAM Serial/Instrument drivers/Traverses/~subVIs/Read_Write_Trav_Config.vi") -> (appended path=w203:path)
            n164 = Build Path(base path=w202, name or relative path=path "ADAM Serial/Instrument drivers/Traverses/~subVIs/DriveConfigGlobal.vi") -> (appended path=w204:path)
            n165 = flat-sequence {
              tunnel: w204 -> [w205]
              tunnel: w203 -> [w207]
              frame #0 {
                n166 = call "Open_Close_Front_Panel.ph.vi"("Front Panel Window:Open"=TRUE, "VI path"=w205) -> ()  [unwired: 2 out]
              }
              frame #1 {
                n167 = call "Open_Close_Front_Panel.ph.vi"("Front Panel Window:Open"=TRUE, "VI path"=w207) -> ()  [unwired: 2 out]
              }
            }
            n168 = event-data() -> ()  [unwired: 1 in, 5 out]
          }
          event Mouse Down? {
            n169 = event-data() -> ()  [unwired: 5 out]
            n170 = global read "Constants_global.vi" "EnFlo SW Folder"() -> (w209:path)
            n171 = Build Path(base path=w209, name or relative path=path "Anemometry/Utilities/Hot_wire_Calculator.vi") -> (appended path=w212:path)
            n172 = call "Open_Close_Front_Panel.ph.vi"("Front Panel Window:Open"=TRUE, "VI path"=w212) -> ()  [unwired: 2 out]
            n173 = event-data() -> ()  [unwired: 1 in, 5 out]
          }
          event Mouse Down? {
            n174 = event-data() -> ()  [unwired: 5 out]
            n175 = global read "Constants_global.vi" "EnFlo SW Folder"() -> (w213:path)
            n176 = Build Path(base path=w213, name or relative path=path "Anemometry/Utilities/Hydrosonic_Manual.vi") -> (appended path=w216:path)
            n177 = call "Open_Close_Front_Panel.ph.vi"("Front Panel Window:Open"=TRUE, "VI path"=w216) -> ()  [unwired: 2 out]
            n178 = event-data() -> ()  [unwired: 1 in, 5 out]
          }
          event Mouse Down? {
            n179 = event-data() -> ()  [unwired: 5 out]
            n180 = global read "Constants_global.vi" "EnFlo SW Folder"() -> (w217:path)
            n181 = Build Path(base path=w217, name or relative path=path "ADAM Client/ADAM client VIs/Fast_FID_Valve_Control.vi") -> (appended path=w220:path)
            n182 = call "Open_Close_Front_Panel.ph.vi"("Front Panel Window:Open"=TRUE, "VI path"=w220) -> ()  [unwired: 2 out]
            n183 = event-data() -> ()  [unwired: 1 in, 5 out]
          }
          event Mouse Down? {
            n184 = event-data() -> ()  [unwired: 5 out]
            n185 = global read "Constants_global.vi" "EnFlo SW Folder"() -> (w221:path)
            n186 = Build Path(base path=w221, name or relative path=path "Anemometry/Utilities/Preference_Panel.vi") -> (appended path=w230:path)
            n187 = Open VI Reference(type specifier VI Refnum (for type only)=refnum<vi> refnum, vi path=w230) -> (vi reference=w223:refnum<vi>, error out=w224:errorcluster)  [unwired: 1 in, 3 out]
            n188 = property class="VI Interface Type 5"(reference=w223, error in=w224, "Front Panel Window:Open"=TRUE) -> (reference out=w226:refnum<vi>, error out=w227:errorcluster)
            n189 = call-by-ref "?"(reference=w226, error in=w227, "Mode"=Preference_Mode."Load, Edit then Save") -> (reference out=w228:refnum<vi>, error out=w229:errorcluster)
            n190 = Close Reference(reference=w228, error in (no error)=w229) -> ()  [unwired: 1 out]
            n191 = event-data("Discard?"=TRUE) -> ()  [unwired: 1 in, 4 out]
          }
          event Mouse Down? {
            n192 = event-data() -> ()  [unwired: 5 out]
            n193 = global read "Constants_global.vi" "EnFlo SW Folder"() -> (w237:path)
            n194 = Build Path(base path=w237, name or relative path=path "ADAM Client/Sub VIs/Gas_Setup.vi") -> (appended path=w244:path)
            n195 = Open VI Reference(type specifier VI Refnum (for type only)=refnum<vi> refnum, vi path=w244) -> (vi reference=w240:refnum<vi>, error out=w241:errorcluster)  [unwired: 1 in, 3 out]
            n196 = property class="VI Interface Type 6"(reference=w240, error in=w241, "Front Panel Window:Open"=TRUE) -> (reference out=w245:refnum<vi>, error out=w243:errorcluster)
            n197 = call-by-ref "?"(reference=w245, error in=w243) -> (reference out=w235:refnum<vi>, error out=w234:errorcluster)  [unwired: 9 in]
            n198 = Close Reference(reference=w235, error in (no error)=w234) -> ()  [unwired: 1 out]
            n199 = event-data("Discard?"=TRUE) -> ()  [unwired: 1 in, 4 out]
          }
          event Mouse Down? {
            n200 = event-data() -> ()  [unwired: 5 out]
            n201 = global read "Constants_global.vi" "EnFlo SW Folder"() -> (w249:path)
            n202 = Build Path(base path=w249, name or relative path=path "ADAM Client/Sub VIs/User_Metadata.vi") -> (appended path=w256:path)
            n203 = Open VI Reference(type specifier VI Refnum (for type only)=refnum<vi> refnum, vi path=w256) -> (vi reference=w252:refnum<vi>, error out=w253:errorcluster)  [unwired: 1 in, 3 out]
            n204 = property class="VI Interface Type 6"(reference=w252, error in=w253, "Front Panel Window:Open"=TRUE) -> (reference out=w257:refnum<vi>, error out=w255:errorcluster)
            n205 = call-by-ref "?"(reference=w257, error in=w255) -> (reference out=w247:refnum<vi>, error out=w246:errorcluster)  [unwired: 9 in]
            n206 = Close Reference(reference=w247, error in (no error)=w246) -> ()  [unwired: 1 out]
            n207 = event-data("Discard?"=TRUE) -> ()  [unwired: 1 in, 4 out]
          }
          event Mouse Down? {
            n208 = event-data() -> ()  [unwired: 5 out]
            n209 = global read "Constants_global.vi" "EnFlo SW Folder"() -> (w263:path)
            n210 = Build Path(base path=w263, name or relative path=path "ADAM Client/Sub VIs/EnFlo_Tunnel_Setup.vi") -> (appended path=w266:path)
            n211 = Open VI Reference(type specifier VI Refnum (for type only)=refnum<vi> refnum, vi path=w266) -> (vi reference=w260:refnum<vi>, error out=w259:errorcluster)  [unwired: 1 in, 3 out]
            n212 = call-by-ref "?"(reference=w260, error in=w259) -> (reference out=w262:refnum<vi>, error out=w261:errorcluster)  [unwired: 9 in]
            n213 = Close Reference(reference=w262, error in (no error)=w261) -> ()  [unwired: 1 out]
            n214 = event-data("Discard?"=TRUE) -> ()  [unwired: 1 in, 4 out]
          }
          event Mouse Down? {
            w277 = TRUE  # Show Panel?
            n215 = event-data() -> ()  [unwired: 5 out]
            n216 = global read "Constants_global.vi" "EnFlo SW Folder"() -> (w272:path)
            n217 = Build Path(base path=w272, name or relative path=path "Anemometry/Anemometry Sub Vis/Gen Trav/Traverse_Space.vi") -> (appended path=w275:path)
            n218 = global read "Trav_pos_global.vi" "Default Traverse Setup"() -> (w267:string)
            n219 = Open VI Reference(type specifier VI Refnum (for type only)=refnum<vi> refnum, vi path=w275) -> (vi reference=w276:refnum<vi>, error out=w268:errorcluster)  [unwired: 1 in, 3 out]
            n220 = call-by-ref "?"(reference=w276, error in=w268, "Show Panel?"=w277, "Traverse Setup"=w267) -> (reference out=w270:refnum<vi>, error out=w269:errorcluster)  [unwired: 8 in, 1 out]
            n221 = Close Reference(reference=w270, error in (no error)=w269) -> ()  [unwired: 1 out]
            n222 = event-data("Discard?"=TRUE) -> ()  [unwired: 1 in, 4 out]
          }
          event Mouse Down? {
            n223 = event-data() -> ()  [unwired: 5 out]
            n224 = global read "Constants_global.vi" "EnFlo SW Folder"() -> (w279:path)
            n225 = Build Path(base path=w279, name or relative path=path "Anemometry/Anemometry Sub Vis/Traverse vi's/EnFlo Tunnel specific/Check_EnFlo_Arm.vi") -> (appended path=w281:path)
            n226 = call "Open_Close_Front_Panel.ph.vi"("Front Panel Window:Open"=TRUE, "VI path"=w281) -> ()  [unwired: 2 out]
            n227 = event-data() -> ()  [unwired: 1 in, 2 out]
          }
          event Mouse Down? {
            n228 = event-data() -> ()  [unwired: 5 out]
            n229 = global read "Constants_global.vi" "EnFlo SW Folder"() -> (w289:path)
            n230 = Build Path(base path=w289, name or relative path=path "Anemometry/Anemometry Sub Vis/Gen Trav/3D_Traverse_move.vi") -> (appended path=w286:path)
            n231 = Strip Path(path=w286) -> (name=w285:string)  [unwired: 1 out]
            n232 = Open VI Reference(vi path=w285) -> (vi reference=w287:refnum<vi>, error out=w288:errorcluster)  [unwired: 1 in, 4 out]
            n233 = property class="VI"(reference=w287, error in=w288) -> (reference out=w283:refnum<vi>, error out=w282:errorcluster, "Front Panel Window:Open"=w284:bool)
            n234 = case shown="False" w284 {
              tunnel: w286 -> [w291 _]
              tunnel: w283 -> [_ w308]
              tunnel: w282 -> [_ w307]
              frame False {
                n235 = global read "Trav_pos_global.vi" "Work in Tunnel Coordinates?"() -> (w301:T46)
                n236 = global read "Trav_pos_global.vi" "Default Traverse Setup"() -> (w299:string)
                n237 = Open VI Reference(type specifier VI Refnum (for type only)=refnum<vi> refnum, vi path=w291) -> (vi reference=w295:refnum<vi>, error out=w296:errorcluster)  [unwired: 1 in, 3 out]
                n238 = property class="VI Interface Type 7"(reference=w295, error in=w296, "Front Panel Window:Open"=TRUE) -> (reference out=w292:refnum<vi>, error out=w293:errorcluster)
                n239 = call-by-ref "?"(reference=w292, error in=w293, "Mode"=Trav_mode."Read traverse position", "Work in Tunnel Coordinates"=w301, "Simulate/Run"=User_Specific_mode."Run VI", "Traverse name"=w299) -> (reference out=w297:refnum<vi>, error out=w298:errorcluster)  [unwired: 9 in, 3 out]
                n240 = Close Reference(reference=w297, error in (no error)=w298) -> ()  [unwired: 1 out]
              }
              frame True {
                n241 = property class="VI"(reference=w308, error in=w307, "Front Panel Window:Open"=TRUE) -> (reference out=w306:refnum<vi>, error out=w305:errorcluster)
                n242 = Close Reference(reference=w306, error in (no error)=w305) -> ()  [unwired: 1 out]
              }
            }
            n243 = event-data() -> ()  [unwired: 1 in, 5 out]
          }
          event Mouse Down? {
            n244 = event-data() -> ()  [unwired: 5 out]
            n245 = Open VI Reference(vi path="Multi_Run_Prog.vi") -> (vi reference=w314:refnum<vi>, error out=w313:errorcluster)  [unwired: 1 in, 4 out]
            n246 = property class="VI"(reference=w314, error in=w313, "Front Panel Window:Open"=TRUE) -> (reference out=w311:refnum<vi>, error out=w312:errorcluster)
            n247 = Close Reference(reference=w311, error in (no error)=w312) -> (error out=w309:errorcluster)
            n248 = Unbundle By Name(w309) -> ("status"=w316:bool)
            n249 = case shown="True" w316 {
              frame False {
              }
              frame True {
                n250 = global read "Constants_global.vi" "EnFlo SW Folder"() -> (w324:path)
                n251 = call "Setup_Filepath.vi"("Setup File Type"=Setup_Filetype."General", "Filename in"="Multi_Run_Filename.txt" ("name or relative path")) -> ("Filename Out"=w317:path)  [unwired: 1 out]
                n252 = Build Path(base path=w324, name or relative path=path "Anemometry/Multi_Run_Prog.vi") -> (appended path=w323:path)
                n253 = call "Read_File_Simple.vi"("Filename"=w317) -> ("string"=w322:string)  [unwired: 2 in, 7 out]
                n254 = String To Path(string=w322) -> (path=w320:path)
                n255 = call "Does_file_exist_(simple).vi"("Pathname"=w320) -> ("exists?"=w321:bool)
                n256 = case shown="False" w321 {
                  tunnel: w323 -> [w326 w338]
                  tunnel: w320 -> [_ w335]
                  frame False {
                    n257 = call "Open_Close_Front_Panel.ph.vi"("Front Panel Window:Open"=TRUE, "VI path"=w326) -> ()  [unwired: 2 out]
                  }
                  frame True {
                    n258 = Open VI Reference(type specifier VI Refnum (for type only)=refnum<vi> refnum, vi path=w338) -> (vi reference=w334:refnum<vi>, error out=w333:errorcluster)  [unwired: 1 in, 3 out]
                    n259 = property class="VI Interface Type 8"(reference=w334, error in=w333, "Front Panel Window:Open"=TRUE) -> (reference out=w331:refnum<vi>, error out=w332:errorcluster)
                    n260 = call-by-ref "?"(reference=w331, error in=w332, "Command filename"=w335, "Setup mode"=T44."Load Command File") -> (reference out=w330:refnum<vi>, error out=w329:errorcluster)  [unwired: 18 in]
                    n261 = Close Reference(reference=w330, error in (no error)=w329) -> ()  [unwired: 1 out]
                  }
                }
              }
            }
            n262 = event-data() -> ()  [unwired: 1 in, 5 out]
          }
          event Mouse Down? {
            w340 = "Calibration.vi" ("name or relative path")
            n263 = event-data() -> ()  [unwired: 5 out]
            n264 = global read "Constants_global.vi" "EnFlo SW Folder"() -> (w346:path)
            n265 = Open VI Reference(vi path=w340) -> (vi reference=w344:refnum<vi>, error out=w343:errorcluster)  [unwired: 1 in, 4 out]
            n266 = Build Path(base path=w346, name or relative path="Anemometry") -> (appended path=w349:path)
            n267 = property class="VI"(reference=w344, error in=w343, "Front Panel Window:Open"=TRUE) -> (reference out=w341:refnum<vi>, error out=w342:errorcluster)
            n268 = Build Path(base path=w349, name or relative path=w340) -> (appended path=w347:path)
            n269 = Close Reference(reference=w341, error in (no error)=w342) -> (error out=w339:errorcluster)
            n270 = Unbundle By Name(w339) -> ("status"=w348:bool)
            n271 = case shown="True" w348 {
              tunnel: w347 -> [_ w351]
              tunnel: w339 -> [_ _]
              frame False {
              }
              frame True {
                n272 = stacked-sequence {
                  seq-local: [w357 _] -> [_ w364]
                  tunnel: w351 -> [_ w365]
                  frame #0 {
                    n273 = call "Setup_Filepath.vi"("Setup File Type"=Setup_Filetype."Calibration Setups", "Filename in"="Current_Setup.xls") -> ("Filename Out"=w352:path)  [unwired: 1 out]
                    n274 = call "Read_File_Simple.vi"("Filename"=w352) -> ("string"=w361:string)  [unwired: 2 in, 7 out]
                    n275 = Format Into String(format string="Calibration Setup File   %s", w352) -> (resulting string=w355:string)  [unwired: 2 in, 1 out]
                    n276 = call "Get_string_subset.vi"("String Name"=w355, "String to split"=w361, "File Label"="Raw data header") -> ("Output string"=w359:string)  [unwired: 1 in, 1 out]
                    n277 = call "Get_Characters_from_string.vi"("Input string"=w359, "Variable name"="Calib filename") -> ("Value"=w358:string)  [unwired: 1 in, 1 out]
                    n278 = call "String_to_Pathname.vi"("Input String"=w358) -> ("path"=w357:path)
                  }
                  frame #1 {
                    n279 = call "Does_file_exist_(simple).vi"("Pathname"=w364) -> ("exists?"=w363:bool)
                    n280 = case shown="True" w363 {
                      tunnel: w365 -> [w366 w381]
                      tunnel: w364 -> [_ w375]
                      frame False {
                        n281 = call "Open_Close_Front_Panel.ph.vi"("Front Panel Window:Open"=TRUE, "VI path"=w366) -> ()  [unwired: 2 out]
                      }
                      frame True {
                        w373 = TRUE ("Front Panel Window:Open")
                        n282 = Open VI Reference(type specifier VI Refnum (for type only)=refnum<vi> refnum, vi path=w381) -> (vi reference=w379:refnum<vi>, error out=w374:errorcluster)  [unwired: 1 in, 3 out]
                        n283 = property class="VI Interface Type 9"(reference=w379, error in=w374, "Front Panel Window:Open"=w373, "Front Panel Window:Auto Center (Deprecated)"=w373) -> (reference out=w378:refnum<vi>, error out=w377:errorcluster)
                        n284 = call-by-ref "?"(reference=w378, error in=w377, "Mode"=Calib_mode."Setup Front Panel", "Calib file"=w375) -> (reference out=w371:refnum<vi>, error out=w370:errorcluster)  [unwired: 15 in, 3 out]
                        n285 = property class="VI Interface Type 9"(reference=w371, error in=w370, "Front Panel Window:Auto Center (Deprecated)"=FALSE ("Front Panel Window:Auto Center")) -> (reference out=w369:refnum<vi>, error out=w368:errorcluster)
                        n286 = Close Reference(reference=w369, error in (no error)=w368) -> ()  [unwired: 1 out]
                      }
                    }
                  }
                }
              }
            }
            n287 = event-data() -> ()  [unwired: 1 in, 5 out]
          }
          event "stop": Mouse Down? {
            n288 = event-data() -> ()  [unwired: 5 out]
            n289 = flat-sequence {
              frame #0 {
                n290 = global write "Dynamic_call_global.ph.vi" "EnFlo Hub running?"(FALSE ("EnFlo Hub running?")) -> ()
              }
              frame #1 {
                n291 = Stop(stop? (T)=TRUE) -> ()
              }
            }
            n292 = event-data() -> ()  [unwired: 1 in, 4 out]
          }
          event "Rig_Control": Value Change {
            n293 = event-data() -> ("OldVal"=w385:cluster{"Ch Name":string, "Boolean":bool}[], "NewVal"=w384:cluster{"Ch Name":string, "Boolean":bool}[])  [unwired: 5 out]
            n294 = for {
              tunnel: w385 -> [w391] mode=indexing
              tunnel: w384 -> [w390] mode=indexing
              n295 = Unbundle By Name(w391) -> ("Ch Name"=w388:string, "Boolean"=w389:bool)
              n296 = Unbundle By Name(w390) -> ("Boolean"=w387:bool)  [unwired: 1 out]
              n297 = Not Equal?(x=w389, y=w387) -> (x != y?=w386:bool)
              n298 = case shown="True" w386 {
                tunnel: w388 -> [_ w393]
                tunnel: w387 -> [_ w400]
                frame False {
                }
                frame True {
                  n299 = Select(t="TRUE", s=w400, f="FALSE") -> (s? t:f=w392:string)
                  n300 = Select(t=1.0, s=w400, f=0.0) -> (s? t:f=w399:dbl)
                  n301 = Format Into String(format string="Are you sure you want to make %s %s?", w393, w392) -> (resulting string=w402:string)  [unwired: 2 in, 1 out]
                  n302 = Format Into String(format string="Make  %s  %s", w393, w392) -> (resulting string=w394:string)  [unwired: 2 in, 1 out]
                  n303 = Two Button Dialog(message=w402, 1:w394, 2:"Cancel" ("T button name (\"OK\")")) -> (T button?=w396:bool)
                  n304 = case shown="False" w396 {
                    tunnel: w393 -> [w407 _]
                    tunnel: w399 -> [w406 _]
                    frame False {
                      n305 = Build Array(w406) -> (w409:dbl[])
                      n306 = Build Array(w407) -> (w408:string[])
                      n307 = call "ASYNC_Adam_client.vi"("Values"=w409, "Channel Names"=w408) -> ()  [unwired: 2 out]
                    }
                    frame True {
                    }
                  }
                }
              }
            }
          }
        }
      }
    }
    "Numeric" <- w8
  }
  n308 = while {
    shift-left: _ -> [w414]
    shift-right: [w415] -> _
    shift-left: "Initialise" -> [w413]
    shift-right: [w416] -> _
    tunnel: "ADAM_Chs_to_Enable.txt" ("name or relative path") -> [w411]
    tunnel: "ADAM_Chs_to_View.txt" ("name or relative path") -> [w410]
    i -> [w412]
    stop <- TRUE continue-if-true
    n309 = case shown="\"Initialise\"" w413 {
      tunnel: ["End" "Initialise" "Wait for call remote sub vi occurrence" "Check type of VI to launch" w486 "Wait until remote sub vi is opened" "Update opened vis array" "Update opened vis array" "Update opened vis array" "Wait until remote sub vi is opened" "Wait for call remote sub vi occurrence"] -> w416
      tunnel: [w418 w431 w436 errorcluster {"status"=FALSE, "code"=0, "source"=""} ("error out") w482 w497 w527 w544 w559 w599 w619] -> w415
      tunnel: w414 -> [w418 w431 w436 _ w482 w497 _ _ _ w599 w619]
      tunnel: w413 -> [w420 _ _ _ _ _ _ _ _ _ _]
      tunnel: w412 -> [_ _ _ _ _ _ _ _ _ _ _]
      tunnel: w411 -> [_ _ w433 _ _ _ _ _ _ _ _]
      tunnel: w410 -> [_ _ w432 _ _ _ _ _ _ _ _]
      frame "No match", Default {
        n310 = Current VI's Path() -> (path=w421:path)
        n311 = Format Into String(format string="The Case\"%s\" was not Matched\nin VI named\n'%s\"" ("Format String"), w420, w421) -> (resulting string=w424:string)  [unwired: 2 in, 1 out]
        n312 = One Button Dialog(message=w424, button name ("OK")="STOP") -> (true=w422:bool)
        n313 = Stop(stop? (T)=w422) -> ()
      }
      frame "Never run" {
        # "These globals are here to make sure they stay in momory\nafter \"Preference Panel\" has finished running"
        n314 = call "Email_With_Log.vi"() -> ()  [unwired: 4 in, 3 out]
        n315 = call "Remember_value.vi"() -> ()  [unwired: 3 in, 1 out]
        n316 = call "Output_Trav_Pos.vi"() -> ()  [unwired: 5 in, 1 out]
        n317 = call "Read_Write_Local_table.vi"() -> ()  [unwired: 3 in, 3 out]
        n318 = call "Overhead_Factor.vi"() -> ()  [unwired: 4 in, 1 out]
        n319 = global read "Trav_pos_global.vi" "Dummy Measurement?"() -> (→"Dummy Measurement":bool)
        n320 = global read "PWAtasksGLOBAL.vi" "Analogue Dev Name"() -> (→"Analogue Dev Name":string)
        n321 = global read "Constants_global.vi" "All_Users"() -> (→"All Users":path)
        n322 = global read "Preference_global.vi" "Rig Setup"() -> (→"Rig Name":string)
      }
      frame "Initialise" {
        n323 = stacked-sequence {
          tunnel: w433 -> [_ _ _ _ w474]
          tunnel: w432 -> [_ _ _ _ w470]
          frame #0 {
            n324 = Generate Occurrence() -> (w457:refnum<k4>)
            n325 = global write "Dynamic_call_global.ph.vi" "Call Remote Subvi"(w457) -> ()
            n326 = Generate Occurrence() -> (w456:refnum<k4>)
            n327 = global write "Dynamic_call_global.ph.vi" "Remote Subvi Opened"(w456) -> ()
            n328 = Initialize Array("", 0) -> (w454:string[])
            n329 = global write "Dynamic_call_global.ph.vi" "Opened VIs"(w454) -> ()
            n330 = global write "Email_transfer_global.vi" "Busy?"(FALSE ("Busy?")) -> ()
            n331 = Current VI's Path() -> (path=w446:path)
            n332 = Strip Path(path=w446) -> (stripped path=w444:path)  [unwired: 1 out]
            n333 = Build Path(base path=w444, name or relative path="Utilities") -> (appended path=w442:path)
            n334 = Build Path(base path=w442, name or relative path="Preference_Panel.vi") -> (appended path=w441:path)
            n335 = Get Date/Time In Seconds() -> (seconds since 1Jan1904=w452:timestamp)
            n336 = To Double Precision Float(number=w452) -> (double precision float=w451:dbl)
            n337 = Open VI Reference(type specifier VI Refnum (for type only)=refnum<vi> refnum, vi path=w441) -> (vi reference=w447:refnum<vi>, error out=w448:errorcluster)  [unwired: 1 in, 3 out]
            n338 = global write "Meas_global.vi" "Start Time of experiment"(w451) -> ()
            n339 = global write "Meas_global.vi" "Post Process"(Post_Process."Post Process Raw Data File" ("Post Process")) -> ()
            n340 = call-by-ref "?"(reference=w447, error in=w448, "Mode"=Preference_Mode."Load Preferences from file") -> (reference out=w449:refnum<vi>, error out=w450:errorcluster)
            n341 = Close Reference(reference=w449, error in (no error)=w450) -> ()  [unwired: 1 out]
          }
          frame #1 {
            w458 = TRUE  # OK
            n342 = call "Get_users_email_addresses.vi"("OK"=w458) -> ()  [unwired: 5 out]
          }
          frame #2 {
            n343 = Current VI's Path() -> (path=w467:path)
            n344 = Open VI Reference(vi path=w467) -> (vi reference=w466:refnum<vi>, error out=w465:errorcluster)  [unwired: 1 in, 4 out]
            n345 = call "Last_modified_date.vi"("Update Now"=TRUE) -> ("RevisionString"=w459:string)  [unwired: 1 out]
            n346 = property class="VI"(reference=w466, error in=w465, "Front Panel Window:Open"=TRUE, "Front Panel Window:Is Frontmost"=FALSE) -> (reference out=w464:refnum<vi>, error out=w463:errorcluster)
            n347 = global write "Meas_global.vi" "ProgRevisionInfo"(w459) -> ()
            n348 = Close Reference(reference=w464, error in (no error)=w463) -> ()  [unwired: 1 out]
          }
          frame #3 {
            n349 = global write "Dynamic_call_global.ph.vi" "EnFlo Hub running?"(TRUE ("EnFlo Hub running?")) -> ()
          }
          frame #4 {
            n350 = global read "Constants_global.vi" "All_Users"() -> (w471:path)
            n351 = Build Path(base path=w471, name or relative path=w470) -> (appended path=w473:path)
            n352 = Build Path(base path=w471, name or relative path=w474) -> (appended path=w476:path)
            n353 = call "Read_File_Simple.vi"("Filename"=w473) -> ("string"=w472:string)  [unwired: 2 in, 7 out]
            n354 = call "Read_File_Simple.vi"("Filename"=w476) -> ("string"=w477:string)  [unwired: 2 in, 7 out]
            n355 = call "Get_array_values_fr_String.vi"("String Value"=w472) -> ("String array"=→"List of ADAM channels to view":string[])  [unwired: 1 out]
            n356 = call "Get_array_values_fr_String.vi"("String Value"=w477) -> ("String array"=→"List of ADAM control channels":string[])  [unwired: 1 out]
          }
        }
        "Iterations" <- 0 ("Iterations")
      }
      frame "Wait for call remote sub vi occurrence" {
        n357 = global read "Dynamic_call_global.ph.vi" "Call Remote Subvi"() -> (w480:refnum<k4>)
        n358 = Wait on Occurrence(2:w480) -> ()  [unwired: 3 out]
      }
      frame "Check type of VI to launch" {
        n359 = global read "Dynamic_call_global.ph.vi" "VI name to launch"() -> (w484:string)
        n360 = Match Pattern(string=w484, regular expression=";") -> (before substring=w481:string, after substring=w483:string)  [unwired: 3 out]
        n361 = case shown="\"Open LDA PWA & An\"" w481 {
          tunnel: ["Open vi" "Open application reference" "Open Analogue input server" w494] -> w486
          tunnel: [w489 w491 w493 w495] -> w485
          tunnel: w484 -> [w489 _ _ _]
          tunnel: w483 -> [_ w491 w493 w495]
          tunnel: w481 -> [_ _ _ w494]
          frame "Other", Default {
          }
          frame "Open Application Reference" {
          }
          frame "Open Analogue Input VI" {
          }
          frame "Open LDA PWA & An" {
          }
        }
        "VI Name" <- w485
      }
      frame "Open application reference" {
        n362 = local read "VI Name"() -> (w498:string)
        n363 = Match Pattern(string=w498, regular expression=";") -> (before substring=w506:string, after substring=w507:string)  [unwired: 3 out]
        n364 = Decimal String To Number(string=w507) -> (number=w508:i32)  [unwired: 3 out]
        n365 = To Unsigned Long Integer(number=w508) -> (unsigned 32bit integer=w505:u32)
        n366 = call "App_Ref_Global.vi"("Mode"=App_Global."Read Global") -> ("Output Array"=w504:T48[])  [unwired: 1 in, 1 out]
        n367 = Open Application Reference(10:w505, 11:w506) -> (0:w499:errorcluster, 3:w503:refnum<vi>)  [unwired: 1 in, 1 out]
        n368 = for {
          tunnel: w504 -> [w510] mode=indexing
          tunnel: w498 -> [w514]
          tunnel: w503 -> [w512]
          tunnel: [w511] -> w502 mode=indexing
          n369 = Unbundle By Name(w510) -> ("Server IP & Port No"=w515:string)
          n370 = Equal?(x=w515, y=w514) -> (x = y?=w513:bool)
          n371 = case shown="False" w513 {
            tunnel: w512 -> [_ w519]
            tunnel: [w516 w518] -> w511
            tunnel: w510 -> [w516 w517]
            frame False {
            }
            frame True {
              n372 = Bundle By Name(cluster=w517, "Application reference"=w519) -> (w518:T48)
            }
          }
        }
        n373 = global write "Dynamic_call_global.ph.vi" "Error Cluster"(w499) -> ()
        n374 = call "App_Ref_Global.vi"("Input Array"=w502, "Mode"=App_Global."Write to Global") -> ()  [unwired: 2 out]
      }
      frame "Open Analogue input server" {
        n375 = local read "VI Name"() -> (w524:string)
        n376 = call "Get_link_info.vi"("VI Name"=w524) -> ("Path name"=w521:path, "Application reference"=w522:refnum<vi>, "Local Call?"=w523:bool)  [unwired: 1 out]
        n377 = global read "Dynamic_call_global.ph.vi" "Analogue Input"() -> (w526:refnum<vi>)
        n378 = case shown="True" w523 {
          tunnel: w526 -> [w532 w536]
          tunnel: [w528 w535] -> w525
          tunnel: [w531 w534] -> w527
          tunnel: w524 -> [w530 _]
          tunnel: w522 -> [w529 _]
          tunnel: w521 -> [_ w533]
          frame False {
            n379 = Open VI Reference(type specifier VI Refnum (for type only)=w532, application reference (local)=w529, vi path=w530) -> (vi reference=w528:refnum<vi>, error out=w531:errorcluster)  [unwired: 1 in, 2 out]
          }
          frame True {
            n380 = Open VI Reference(type specifier VI Refnum (for type only)=w536, vi path=w533) -> (vi reference=w535:refnum<vi>, error out=w534:errorcluster)  [unwired: 1 in, 3 out]
          }
        }
        n381 = global write "Dynamic_call_global.ph.vi" "Analogue Input"(w525) -> ()
      }
      frame "Open LDA PWA & An" {
        n382 = local read "VI Name"() -> (w541:string)
        n383 = call "Get_link_info.vi"("VI Name"=w541) -> ("Path name"=w538:path, "Application reference"=w539:refnum<vi>, "Local Call?"=w540:bool)  [unwired: 1 out]
        n384 = global read "Dynamic_call_global.ph.vi" "Take LDA PWA & An"() -> (w543:refnum<vi>)
        n385 = case shown="True" w540 {
          tunnel: w543 -> [w549 w553]
          tunnel: [w545 w552] -> w542
          tunnel: [w548 w551] -> w544
          tunnel: w541 -> [w547 _]
          tunnel: w539 -> [w546 _]
          tunnel: w538 -> [_ w550]
          frame False {
            n386 = Open VI Reference(type specifier VI Refnum (for type only)=w549, application reference (local)=w546, vi path=w547) -> (vi reference=w545:refnum<vi>, error out=w548:errorcluster)  [unwired: 1 in, 2 out]
          }
          frame True {
            n387 = Open VI Reference(type specifier VI Refnum (for type only)=w553, vi path=w550) -> (vi reference=w552:refnum<vi>, error out=w551:errorcluster)  [unwired: 1 in, 3 out]
          }
        }
        n388 = global write "Dynamic_call_global.ph.vi" "Take LDA PWA & An"(w542) -> ()
      }
      frame "Open vi" {
        n389 = local read "VI Name"() -> (w558:string)
        n390 = call "Get_link_info.vi"("VI Name"=w558) -> ("Path name"=w557:path, "Application reference"=w556:refnum<vi>, "Local Call?"=w555:bool)  [unwired: 1 out]
        n391 = case shown="\"No Match\", Default" w558 {
          tunnel: [w560 w569 w581] -> w559
          tunnel: w558 -> [w565 w568 w585]
          tunnel: w557 -> [_ _ w582]
          tunnel: w556 -> [_ w567 w584]
          tunnel: w555 -> [_ w566 w583]
          frame "No Match", Default {
            n392 = Format Into String(format string="VI named \"%s\" Not matched" ("Format String"), w565) -> (resulting string=w562:string)  [unwired: 2 in, 1 out]
            n393 = Bundle By Name(cluster=errorcluster {"status"=FALSE, "code"=0, "source"=""} ("error out"), "source"=w562, "status"=TRUE ("Bundle Element")) -> (w560:errorcluster)
          }
          frame "Program_Active_server.vi" {
            n394 = global read "Dynamic_call_global.ph.vi" "Program Active server"() -> (w571:refnum<vi>)
            n395 = case shown="True" w566 {
              tunnel: w571 -> [w576 w580]
              tunnel: [w575 w579] -> w570
              tunnel: [w574 w578] -> w569
              tunnel: w568 -> [w573 w577]
              tunnel: w567 -> [w572 _]
              frame False {
                n396 = Open VI Reference(type specifier VI Refnum (for type only)=w576, application reference (local)=w572, vi path=w573) -> (vi reference=w575:refnum<vi>, error out=w574:errorcluster)  [unwired: 1 in, 2 out]
              }
              frame True {
                n397 = Open VI Reference(type specifier VI Refnum (for type only)=w580, vi path=w577) -> (vi reference=w579:refnum<vi>, error out=w578:errorcluster)  [unwired: 1 in, 3 out]
              }
            }
            n398 = global write "Dynamic_call_global.ph.vi" "Program Active server"(w570) -> ()
          }
          frame "GPIB_Server.vi" {
            n399 = global read "Dynamic_call_global.ph.vi" "GPIB_Server.vi"() -> (w587:refnum<vi>)
            n400 = case shown="False" w583 {
              tunnel: w587 -> [w592 w596]
              tunnel: [w591 w595] -> w586
              tunnel: [w590 w594] -> w581
              tunnel: w585 -> [w588 _]
              tunnel: w584 -> [w589 _]
              tunnel: w582 -> [_ w593]
              frame False {
                n401 = Open VI Reference(type specifier VI Refnum (for type only)=w592, application reference (local)=w589, vi path=w588) -> (vi reference=w591:refnum<vi>, error out=w590:errorcluster)  [unwired: 1 in, 2 out]
              }
              frame True {
                n402 = Open VI Reference(type specifier VI Refnum (for type only)=w596, vi path=w593) -> (vi reference=w595:refnum<vi>, error out=w594:errorcluster)  [unwired: 1 in, 3 out]
              }
            }
            n403 = global write "Dynamic_call_global.ph.vi" "GPIB_Server.vi"(w586) -> ()
          }
        }
      }
      frame "Update opened vis array" {
        w601 = TRUE  # Dialog Box
        n404 = local read "VI Name"() -> (w600:string)
        n405 = Unbundle By Name(w599) -> ("status"=w604:bool, "source"=w602:string)
        n406 = case shown="True" w604 {
          tunnel: w599 -> [w606 w615]
          tunnel: [w606 w614] -> w603
          tunnel: w600 -> [w607 w610]
          tunnel: w602 -> [_ w613]
          frame False {
            n407 = global read "Dynamic_call_global.ph.vi" "Opened VIs"() -> (w608:string[])
            n408 = To Upper Case(1:w607) -> (0:w605:string)
            n409 = Build Array (concatenate)(w608, w605) -> (w609:string[])
            n410 = global write "Dynamic_call_global.ph.vi" "Opened VIs"(w609) -> ()
          }
          frame True {
            n411 = Concatenate Strings(w610, " " ("Substring"), w613) -> (w611:string)
            n412 = Bundle By Name(cluster=w615, "source"=w611) -> (w614:errorcluster)
          }
        }
        n413 = call "EnFlo_Error_Handler.vi"("error in (no error)"=w603, "Error Type"="Dynamic Call", "Dialog Box (T)"=w601) -> ()  [unwired: 3 out]
      }
      frame "Wait until remote sub vi is opened" {
        n414 = global read "Dynamic_call_global.ph.vi" "Remote Subvi Opened"() -> (w620:refnum<k4>)
        n415 = local read "Iterations"() -> (w618:i32)
        n416 = Increment(x=w618) -> (x+1=w617:i32)
        n417 = local write "Iterations"(w617) -> ()
        n418 = Set Occurrence(w620) -> ()
      }
    }
  }
  n419 = while {
    i -> [w621]
    stop <- FALSE stop-if-true
    n420 = stacked-sequence {
      tunnel: w621 -> [_ w666]
      frame #0 {
        n421 = global read "Dynamic_call_global.ph.vi" "EnFlo Hub running?"() -> (w625:bool)
        n422 = Equal?(x="Tab Control", y=T1."Adam Table" ("Tab Control")) -> (x = y?=w626:bool)
        n423 = And(x=w626, y=w625) -> (x .and. y?=w624:bool)
        n424 = case shown="False" w624 {
          frame True {
            n425 = local read "List of ADAM channels to view"() -> (w635:string[])
            n426 = local read "List of ADAM control channels"() -> (w638:string[])
            n427 = Build Array (concatenate)(w638, w635) -> (w637:string[])
            n428 = call "Get_Current_Scan_client.vi"("ADAM Ch Names"=w637) -> ("Ch Description Array"=w632:T50[], "Numerical Values"=w636:dbl[])  [unwired: 2 out]
            n429 = Array Size(array=w638) -> (size(s)=w633:i32)
            n430 = Array Subset(array=w632, index=w633) -> (w631:T50[])  [unwired: 1 in]
            n431 = Array Subset(array=w636, index=w633) -> (w630:dbl[])  [unwired: 1 in]
            n432 = for {
              tunnel: w631 -> [w645] mode=indexing
              tunnel: [w644] -> w629 mode=indexing
              tunnel: cluster{"Ch Name":string, "Numeric":dbl} {"Ch Name"="", "Numeric"=0.0} ("Cluster") -> [w643]
              tunnel: w630 -> [w641] mode=indexing
              n433 = Unbundle By Name(w645) -> ("Ch Name"=w642:string)
              n434 = Bundle By Name(cluster=w643, "Ch Name"=w642, "Numeric"=w641) -> (w644:cluster{"Ch Name":string, "Numeric":dbl})
            }
            "Current Values" <- w629
            n435 = for {
              N: w633 -> [_]
              tunnel: cluster{"Ch Name":string, "Boolean":bool} {"Ch Name"="", "Boolean"=FALSE} ("Cluster") -> [w652]
              tunnel: w632 -> [w651] mode=indexing
              tunnel: w636 -> [w649] mode=indexing
              tunnel: [w646] -> w639 mode=indexing
              n436 = Unbundle By Name(w651) -> ("Ch Name"=w650:string)
              n437 = Greater?(x=w649, y=0.5) -> (0:w647:bool)
              n438 = Bundle By Name(cluster=w652, "Ch Name"=w650, "Boolean"=w647) -> (w646:cluster{"Ch Name":string, "Boolean":bool})
            }
            n439 = local write "Rig_Control"(w639) -> ()
          }
          frame False {
          }
        }
      }
      frame #1 {
        w664 = 300 ("y")
        n440 = Quotient & Remainder(x=w666, y=3600) -> (x-y*floor(x/y)=w667:i32)  [unwired: 1 out]
        n441 = Quotient & Remainder(x=w666, y=900) -> (x-y*floor(x/y)=w663:i32)  [unwired: 1 out]
        n442 = Equal?(x=w667, y=w664) -> (x = y?=w661:bool)
        n443 = Equal?(x=w664, y=w663) -> (x = y?=w662:bool)
        n444 = Or(x=w661, y=w662) -> (x .or. y?=w654:bool)
        n445 = Select(t=3 ("Months of History to backup"), s=w661, f=0) -> (s? t:f=w658:i32)
        n446 = global read "Preference_global.vi" "Server Comms"() -> (w656:T49)
        n447 = Equal?(x=w656, y=Server_Comms."Server Link Healthy" ("Server Comms")) -> (x = y?=w655:bool)
        n448 = And(x=w654, y=w655) -> (x .and. y?=w653:bool)
        n449 = case shown="True" w653 {
          tunnel: w658 -> [_ w671]
          frame False {
          }
          frame True {
            w669 = TRUE  # Check Updates on Server?
            w670 = TRUE  # Get all Server Files
            n450 = call "Backup_Client.vi"("Check Updates on Server?"=w669, "Get all Server Files"=w670, "Months of History to backup"=w671) -> ()  [unwired: 1 out]
          }
        }
      }
    }
    n451 = Wait (ms)(milliseconds to wait=u32 1000) -> ()  [unwired: 1 out]
  }
